vi "Drop Message Core.vi"(11 "Create Ref Message in":refnum<class "Create Ref Message.lvclass">) -> ()   [LabVIEW 2020, in "Create Ref Message.lvclass"]
doc: "(<B>Filename</B>: Actor Framework.lvlib:Message.lvclass:Drop Message Core.vi)\n\nDefines what a message does if it is in the message queue when the queue is released. At this point, the actor has shut down, so it will never process the message.\n\nBy default, this method does nothing. A child class may override it to define behavior. National Instruments provides the Reply Msg class to override this method. This class releases its internal queue, which causes any caller of the Send Message and Wait For Response method to stop waiting and return an error."
uses:
  <vilib>/gpm_packages/@cs/Network-interface/Source/Create Ref Message/Create Ref Message.lvclass
  <vilib>/gpm_packages/@cs/Network-interface/Source/Create Ref Message/Create Ref Message.lvclass/Create Ref Message.ctl
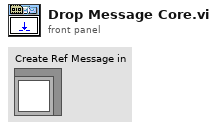
[diagram p1: front panel]
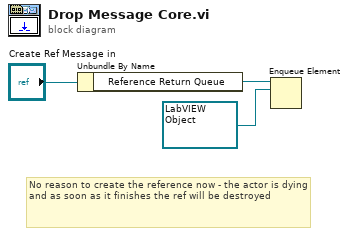
[diagram p0: block diagram]
diagram:
  # "No reason to create the reference now - the actor is dying and as soon as it finishes the ref will be destroyed"
  n1 = Unbundle By Name("Create Ref Message in") -> ("Reference Return Queue"=w2:refnum<queue>)
  n2 = Enqueue Element(queue=w2, element=refnum<data-value> refnum) -> ()  [unwired: 2 in, 3 out]
